vi "Sensirion SHT25 - VISA read humidity.vi"(8 "Error In":errorcluster, 11 "VISA in":refnum<visa-resource-name>) -> (0 "Error Out":errorcluster, 1 "humidity":dbl, 3 "VISA out":refnum<visa-resource-name>)   [LabVIEW 2012]
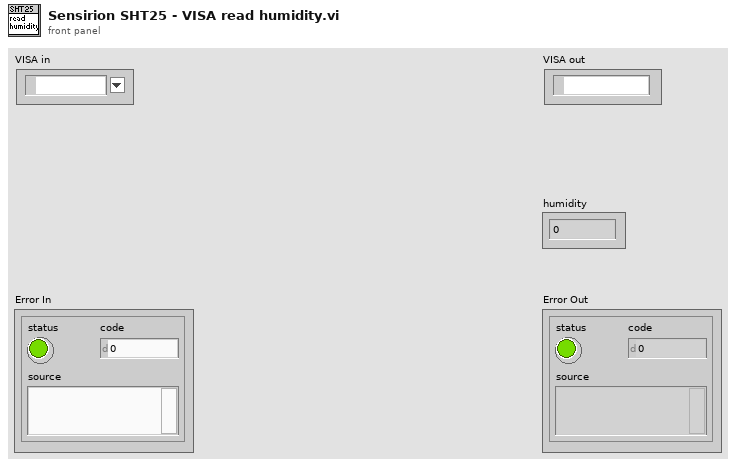
[diagram p1: front panel]
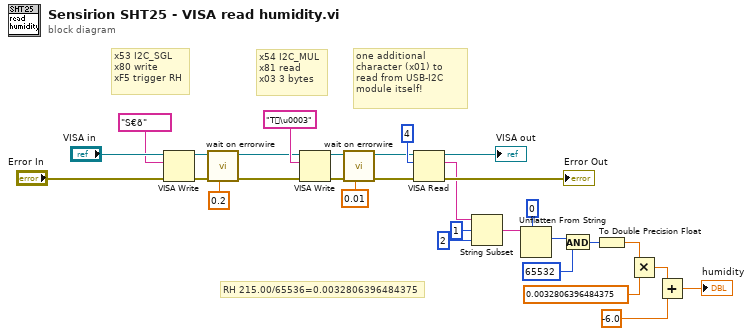
[diagram p0: block diagram]
diagram:
  # "RH 215.00/65536=0.0032806396484375"
  # "one additional character (x01) to read from USB-I2C module itself!"
  # "x54 I2C_MUL\nx81 read\nx03 3 bytes"
  # "x53 I2C_SGL\nx80 write\nxF5 trigger RH"
  n1 = VISA Write(VISA resource name="VISA in", write buffer="S€õ", error in (no error)="Error In") -> (VISA resource name out=w21:refnum<visa-resource-name>, error out=w23:errorcluster)  [unwired: 1 out]
  n2 = call "wait on errorwire.vi"("Delay Time (s)"=0.2, "error in (no error)"=w23) -> ("error out"=w20:errorcluster)  [unwired: 9 in]
  n3 = VISA Write(VISA resource name=w21, write buffer="T\u0003", error in (no error)=w20) -> (VISA resource name out=w18:refnum<visa-resource-name>, error out=w16:errorcluster)  [unwired: 1 out]
  n4 = call "wait on errorwire.vi"("Delay Time (s)"=0.01, "error in (no error)"=w16) -> ("error out"=w15:errorcluster)  [unwired: 9 in]
  n5 = VISA Read(VISA resource name=w18, byte count=u32 4, error in (no error)=w15) -> (VISA resource name out=→"VISA out":refnum<visa-resource-name>, read buffer=w2:string, error out=→"Error Out":errorcluster)  [unwired: 1 out]
  n6 = String Subset(string=w2, offset (0)=1, length (rest)=2 ("length (rest)")) -> (substring=w1:string)
  n7 = Unflatten From String(type=u16 0, binary string=w1) -> (value=w10:u16)  [unwired: 3 in, 2 out]
  n8 = And(x=w10, y=u16 65532) -> (x .and. y?=w6:u16)
  n9 = To Double Precision Float(number=w6) -> (double precision float=w11:dbl)
  n10 = Multiply(x=w11, y=0.0032806396484375) -> (x*y=w8:dbl)
  n11 = Add(x=w8, y=-6.0) -> (x+y=→"humidity":dbl)
